vi "TrimAlpha.vi"(11 "input cluster":T1) -> (3 "output cluster":T1)   [LabVIEW 2014]
uses:
  <vilib>/picture/picture.llb/imagedata.ctl
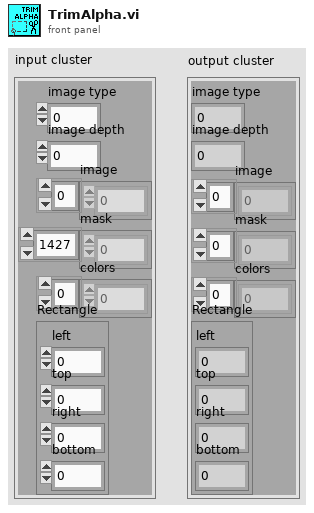
[diagram p1: front panel]
types:
  T1 = typedef "imagedata.ctl" = cluster{"image type":i32, "image depth":i32, "image":u8[], "mask":u8[], "colors":u32[], "Rectangle":cluster{"left":i16, "top":i16, "right":i16, "bottom":i16}}
  T2 = cluster{"left":i16, "top":i16, "right":i16, "bottom":i16}
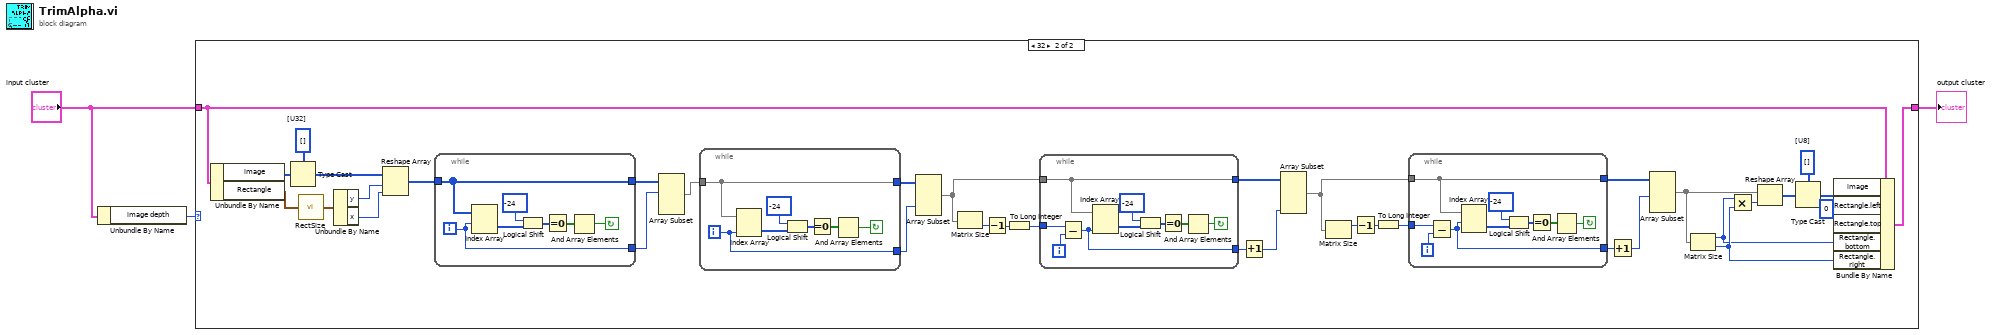
[diagram p0: block diagram]
diagram:
  n1 = Unbundle By Name("input cluster") -> ("image depth"=w3:i32)
  n2 = case shown="32" w3 {
    tunnel: "input cluster" -> [w4 w13]
    tunnel: [w4 w5] -> w1
    frame Default {
    }
    frame 32 {
      w8 = i16 0 ("Rectangle.left")
      w9 = u8[] []  # [U8]
      w40 = u32[] []  # [U32]
      n3 = Unbundle By Name(w13) -> ("image"=w41:u8[], "Rectangle"=w38:T2)
      n4 = Type Cast(type=w40, x=w41) -> (*(type *) &x=w37:u32[])
      n5 = call <vilib>:"RectSize.vi"("rect"=w38) -> ("point"=w39:cluster{"x":i16, "y":i16})
      n6 = Unbundle By Name(w39) -> ("y"=w32:i16, "x"=w36:i16)
      n7 = Reshape Array(w37, w32, w36) -> (w33:u32[][])
      n8 = while {
        tunnel: [w68] -> w30
        tunnel: w33 -> [w67]
        tunnel: [w67] -> w31
        i -> [w68]
        stop <- w69 continue-if-true
        n9 = Index Array(array=w67, index (row)=w68) -> (element=w73:u32[])  [unwired: 1 in]
        n10 = Logical Shift(y=i16 -24, x=w73) -> (x << y=w71:u32[])
        n11 = Equal To 0?(x=w71) -> (x = 0?=w70:bool[])
        n12 = And Array Elements(Boolean array=w70) -> (logical AND=w69:bool)
      }
      n13 = Array Subset(array=w31, index (row)=w30) -> (w29:u32[][])  [unwired: 3 in]
      n14 = while {
        tunnel: w29 -> [w60]
        tunnel: [w61] -> w27
        tunnel: [w60] -> w28
        i -> [w61]
        stop <- w62 continue-if-true
        n15 = Index Array(array=w60, index (col)=w61) -> (element=w66:u32[])  [unwired: 1 in]
        n16 = Logical Shift(y=i16 -24, x=w66) -> (x << y=w64:u32[])
        n17 = Equal To 0?(x=w64) -> (x = 0?=w63:bool[])
        n18 = And Array Elements(Boolean array=w63) -> (logical AND=w62:bool)
      }
      n19 = Array Subset(array=w28, index (col)=w27) -> (w26:u32[][])  [unwired: 3 in]
      n20 = Matrix Size(0:w26) -> (2:w25:i32)  [unwired: 1 out]
      n21 = Decrement(x=w25) -> (x-1=w35:i32)
      n22 = To Long Integer(number=w35) -> (32bit integer=w34:i32)
      n23 = while {
        tunnel: w26 -> [w52]
        tunnel: w34 -> [w54]
        tunnel: [w51] -> w23
        tunnel: [w52] -> w24
        i -> [w53]
        stop <- w55 continue-if-true
        n24 = Subtract(x=w54, y=w53) -> (x-y=w51:i32)
        n25 = Index Array(array=w52, index (col)=w51) -> (element=w59:u32[])  [unwired: 1 in]
        n26 = Logical Shift(y=i16 -24, x=w59) -> (x << y=w57:u32[])
        n27 = Equal To 0?(x=w57) -> (x = 0?=w56:bool[])
        n28 = And Array Elements(Boolean array=w56) -> (logical AND=w55:bool)
      }
      n29 = Increment(x=w23) -> (x+1=w15:i32)
      n30 = Array Subset(array=w24, length (col)=w15) -> (w16:u32[][])  [unwired: 3 in]
      n31 = Matrix Size(0:w16) -> (1:w17:i32)  [unwired: 1 out]
      n32 = Decrement(x=w17) -> (x-1=w18:i32)
      n33 = To Long Integer(number=w18) -> (32bit integer=w19:i32)
      n34 = while {
        tunnel: w16 -> [w43]
        tunnel: w19 -> [w45]
        tunnel: [w42] -> w21
        tunnel: [w43] -> w20
        i -> [w44]
        stop <- w46 continue-if-true
        n35 = Subtract(x=w45, y=w44) -> (x-y=w42:i32)
        n36 = Index Array(array=w43, index (row)=w42) -> (element=w50:u32[])  [unwired: 1 in]
        n37 = Logical Shift(y=i16 -24, x=w50) -> (x << y=w48:u32[])
        n38 = Equal To 0?(x=w48) -> (x = 0?=w47:bool[])
        n39 = And Array Elements(Boolean array=w47) -> (logical AND=w46:bool)
      }
      n40 = Increment(x=w21) -> (x+1=w22:i32)
      n41 = Array Subset(array=w20, length (row)=w22) -> (w12:u32[][])  [unwired: 3 in]
      n42 = Matrix Size(0:w12) -> (1:w6:i32, 2:w7:i32)
      n43 = Multiply(x=w6, y=w7) -> (x*y=w14:i32)
      n44 = Reshape Array(w12, w14) -> (w11:u32[])
      n45 = Type Cast(type=w9, x=w11) -> (*(type *) &x=w10:u8[])
      n46 = Bundle By Name(cluster=w13, "image"=w10, "Rectangle.left"=w8, "Rectangle.top"=w8, "Rectangle.bottom"=w6, "Rectangle.right"=w7) -> (w5:T1)
    }
  }
  "output cluster" <- w1
